vi "Convolution PtByPt.vi"(0 "x":dbl format="%0.2f", 1 "sample length x":i32=100, 2 "y":dbl format="%0.2f", 3 "sample length y":i32=100, 4 "initialize":bool) -> (5 "X*Y":dbl[](array[numeric]), 6 "error":i32)   [LabVIEW 2017, in "NI_PtbyPt.lvlib"]
doc: "Computes the convolution of <B>x</B> and <B>y</B>."
uses:
  <vilib>/ptbypt/NI_PtbyPt.lvlib
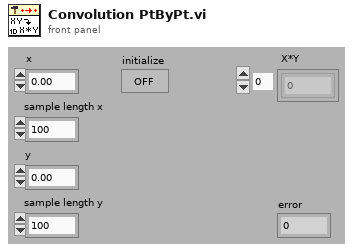
[diagram p1: front panel]
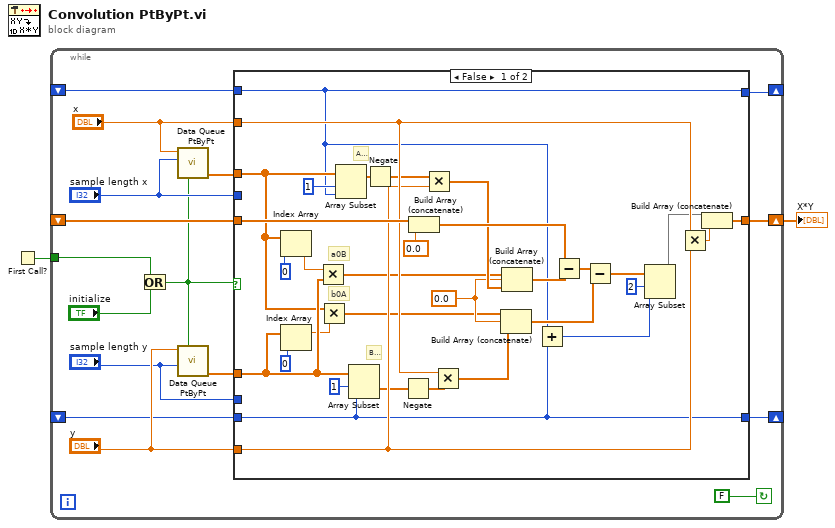
[diagram p0: block diagram]
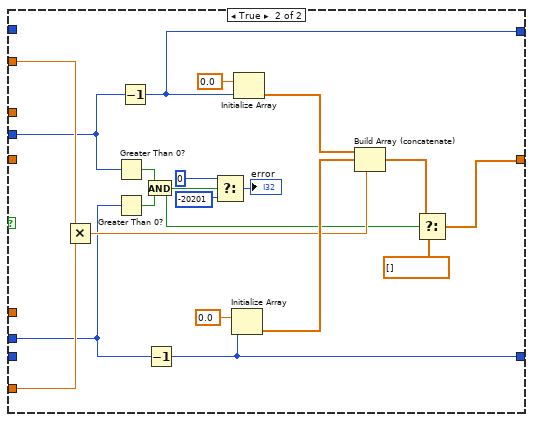
[diagram p2: hidden frame]
diagram:
  n1 = First Call?() -> (First Call?: T/F=w1:bool)
  n2 = while {
    tunnel: w1 -> [w5]
    shift-left: _ -> [w7]
    shift-right: [w8] -> _
    shift-left: _ -> [w9]
    shift-right: [w10] -> _
    shift-left: _ -> [w17]
    shift-right: [w18] -> w2
    stop <- FALSE continue-if-true
    n3 = Or(x=w5, y="initialize") -> (x .or. y?=w3:bool)
    n4 = call <vilib>:"Data Queue PtByPt.vi"("initialize"=w3, "sample length"="sample length x", "input data point"="x") -> ("Previous Queue"=w15:dbl[])  [unwired: 4 in, 4 out]
    n5 = call <vilib>:"Data Queue PtByPt.vi"("initialize"=w3, "sample length"="sample length y", "input data point"="y") -> ("Previous Queue"=w16:dbl[])  [unwired: 4 in, 4 out]
    n6 = case shown="False" w3 {
      tunnel: [w51 w53] -> w18
      tunnel: w17 -> [w50 _]
      tunnel: w16 -> [w49 _]
      tunnel: w15 -> [w48 _]
      tunnel: "sample length x" -> [_ w61]
      tunnel: "x" -> [w47 w71]
      tunnel: "y" -> [w46 w70]
      tunnel: "sample length y" -> [_ w62]
      tunnel: [w20 w64] -> w10
      tunnel: w9 -> [w20 _]
      tunnel: [w19 w63] -> w8
      tunnel: w7 -> [w19 _]
      frame False {
        w23 = 0.0 ("Input Element")
        # "b0A"
        # "a0B"
        # "B--"
        # "A--"
        n7 = Index Array(array=w48, index=0 ("Index")) -> (element=w30:dbl)
        n8 = Index Array(array=w49, index=0 ("Index")) -> (element=w32:dbl)
        n9 = Multiply(x=w30, y=w49) -> (x*y=w24:dbl[])
        n10 = Multiply(x=w48, y=w32) -> (x*y=w22:dbl[])
        n11 = Array Subset(array=w48, index=1 ("Array Index"), length=w20) -> (w37:dbl[])
        n12 = Array Subset(array=w49, index=1 ("Array Index"), length=w19) -> (w36:dbl[])
        n13 = Negate(x=w37) -> (-x=w27:dbl[])
        n14 = Negate(x=w36) -> (-x=w26:dbl[])
        n15 = Build Array (concatenate)(w50, 0.0 ("Input Element")) -> (w44:dbl[])
        n16 = Multiply(x=w27, y=w46) -> (x*y=w35:dbl[])
        n17 = Multiply(x=w47, y=w26) -> (x*y=w29:dbl[])
        n18 = Build Array (concatenate)(w22, w23, w29) -> (w28:dbl[])
        n19 = Build Array (concatenate)(w24, w23, w35) -> (w34:dbl[])
        n20 = Add(x=w20, y=w19) -> (x+y=w21:i32)
        n21 = Subtract(x=w44, y=w34) -> (x-y=w43:dbl[])
        n22 = Subtract(x=w43, y=w28) -> (x-y=w25:dbl[])
        n23 = Array Subset(array=w25, index=2 ("Array Index"), length=w21) -> (w41:dbl[])
        n24 = Multiply(x=w47, y=w46) -> (x*y=w40:dbl)
        n25 = Build Array (concatenate)(w41, w40) -> (w51:dbl[])
      }
      frame True {
        n26 = Multiply(x=w71, y=w70) -> (x*y=w65:dbl)
        n27 = Greater Than 0?(x=w61) -> (x > 0?=w60:bool)
        n28 = Greater Than 0?(x=w62) -> (x > 0?=w59:bool)
        n29 = Decrement(x=w61) -> (x-1=w64:i32)
        n30 = And(x=w60, y=w59) -> (x .and. y?=w58:bool)
        n31 = Decrement(x=w62) -> (x-1=w63:i32)
        n32 = Select(t=0, s=w58, f=-20201) -> (s? t:f=→"error":i32)
        n33 = Initialize Array(0.0 ("Element Data"), w63) -> (w68:dbl[])
        n34 = Initialize Array(0.0 ("Element Data"), w64) -> (w66:dbl[])
        n35 = Build Array (concatenate)(w66, w68, w65) -> (w54:dbl[])
        n36 = Select(t=w54, s=w58, f=dbl[] []) -> (s? t:f=w53:dbl[])
      }
    }
  }
  "X*Y" <- w2
